vi "Init.vi"(7 "Enclave":refnum<class "Enclave.lvclass">, 8 "error in (no error)":errorcluster, 11 "Event":refnum<user-event>) -> (0 "error out":errorcluster, 3 "Event out":refnum<class "Event.lvclass">)   [LabVIEW 2022 SP3, in "Enclave.lvlib" / "Event.lvclass"]
uses:
  Event.lvclass
  Enclave Event.ctl
  Element.ctl
  Enclave/Enclave.lvclass
  Event.lvclass/Event.ctl
  Enclave.lvlib
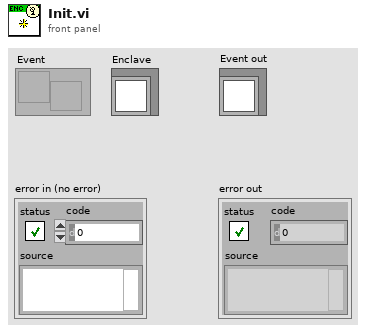
[diagram p1: front panel]
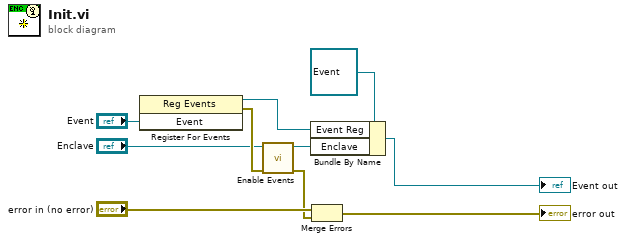
[diagram p0: block diagram]
diagram:
  n1 = register-events("Event") -> (reference out=w3:refnum<event-registration>, error out=w10:errorcluster)  [unwired: 2 in]
  n2 = call "Enable Events.vi"("error in (no error)"=w10, "Enclave in"="Enclave") -> ("error out"=w1:errorcluster, "Enclave out"=w4:refnum<class "Enclave.lvclass">)  [unwired: 8 in]
  n3 = Bundle By Name(cluster=refnum<class "Event.lvclass"> refnum ("Event in"), "Event Reg"=w3, "Enclave"=w4) -> (→"Event out":refnum<class "Event.lvclass">)
  n4 = Merge Errors("error in (no error)", w1) -> (→"error out":errorcluster)
